vi "Format TBM.vi"(4 "WorkTable":refnum<class "WorkTable Class.lvclass">, 6 "Bond Pad Groups":T1[](array[typedef]), 7 "Inner/Outer":string, 8 "error in":errorcluster, 9 "Slot":i32, 10 "Chuck":i32, 11 "Console Log in":refnum<class "Console Log.lvclass">) -> (0 "error out":errorcluster, 2 "Formatted TBM":string[](array[string]), 3 "Console Log out":refnum<class "Console Log.lvclass">)   [LabVIEW 2011, in "Console Log.lvclass"]
uses:
  Console Log.lvclass
  Shared Components/Utils/Type Definitions/3d Line.ctl
  Shared Components/Vec3d Class/Vec3d Class.lvclass
  Shared Components/WorkTable Class/WorkTable Class.lvclass
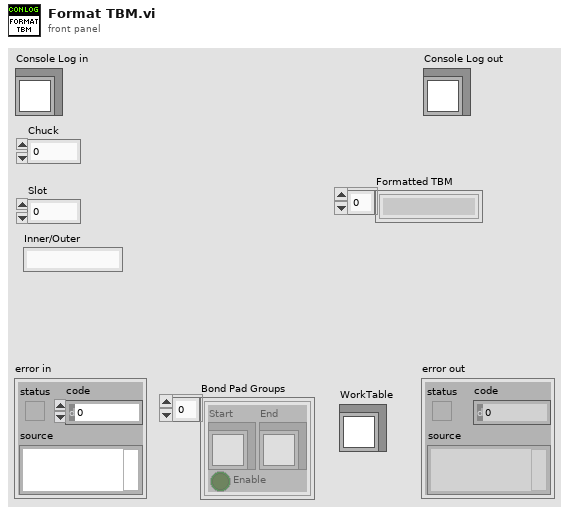
[diagram p1: front panel]
types:
  T1 = typedef "3d Line.ctl" = cluster{"Start":refnum<class "Vec3d Class.lvclass">, "End":refnum<class "Vec3d Class.lvclass">, "Enable":bool}
  T2 = typedef "Worktable_Module Slot.ctl" = cluster{"Slot State":enum16{"Empty", "Unglued", "Stamped", "PartOnTop", "Weighted", "Unpotted", "Potted"}, "BBM Type":enum16{"None", "BBM", "GlassSlide"}, "HDI Type":enum16{"None", "HDI", "Polyimide"}, "Vacuum Channel":u8, "Location/Orientation BBM":T3, "Location/Orientation HDI":T3, "S/N":string}
  T3 = typedef "Position_Orientation.ctl" = cluster{"Center":refnum<class "Vec3d Class.lvclass">, "Orientation":refnum<class "Orient3d Class.lvclass">}
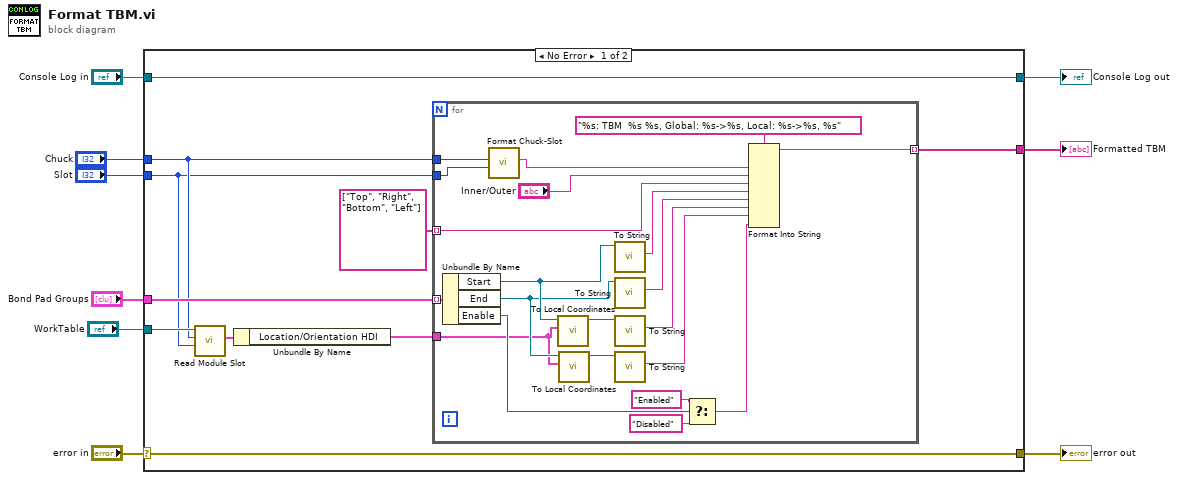
[diagram p0: block diagram]
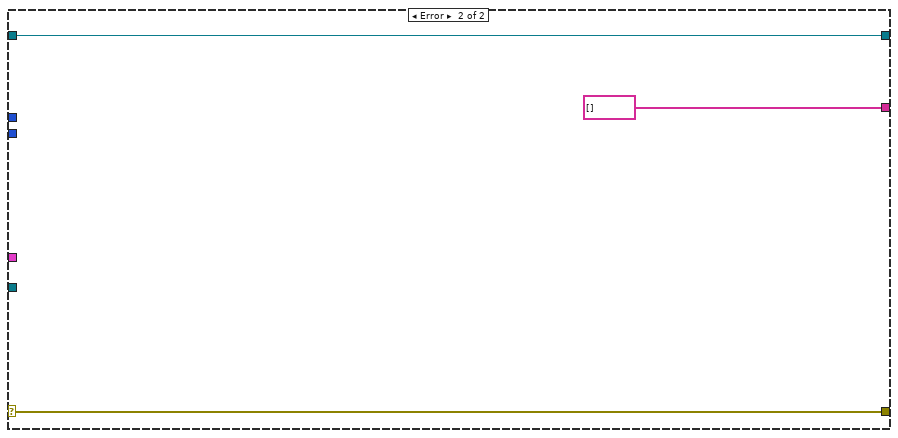
[diagram p2: hidden frame]
diagram:
  n1 = case shown="No Error" "error in" {
    selector: "error in" -> [w18 w43]
    tunnel: [w18 w43] -> w8
    tunnel: [w19 w42] -> w6
    tunnel: "Console Log in" -> [w19 w42]
    tunnel: "Bond Pad Groups" -> [w17 _]
    tunnel: [w16 string[] []] -> w4
    tunnel: "Chuck" -> [w13 _]
    tunnel: "Slot" -> [w12 _]
    tunnel: "WorkTable" -> [w14 _]
    frame No Error {
      n2 = call-dynamic "Read Module Slot.vi"("slot"=w12, "chuck"=w13, "WorkTable in"=w14) -> ("Module Slot"=w11:T2)  [unwired: 6 in, 2 out]
      n3 = Unbundle By Name(w11) -> ("Location/Orientation HDI"=w10:T3)
      n4 = for {
        tunnel: w17 -> [w40] mode=indexing
        tunnel: [w33] -> w16 mode=indexing
        tunnel: string[] ["Top", "Right", "Bottom", "Left"] -> [w31] mode=indexing
        tunnel: w13 -> [w22]
        tunnel: w12 -> [w21]
        tunnel: w10 -> [w23]
        n5 = Unbundle By Name(w40) -> ("Start"=w25:refnum<class "Vec3d Class.lvclass">, "End"=w24:refnum<class "Vec3d Class.lvclass">, "Enable"=w39:bool)
        n6 = call "Format Chuck-Slot.vi"("Slot"=w21, "Chuck"=w22) -> ("Formatted Chuck/Slot"=w20:string)  [unwired: 7 in, 2 out]
        n7 = call "To Local Coordinates.vi"("Center/Orientation"=w23, "Global Coordinates"=w25) -> ("Local Coordinates"=w30:refnum<class "Vec3d Class.lvclass">)  [unwired: 8 in, 1 out]
        n8 = call "To Local Coordinates.vi"("Center/Orientation"=w23, "Global Coordinates"=w24) -> ("Local Coordinates"=w29:refnum<class "Vec3d Class.lvclass">)  [unwired: 8 in, 1 out]
        n9 = call "To String.vi"("Vec3d in"=w25) -> ("Vec3d String"=w35:string)  [unwired: 8 in, 2 out]
        n10 = call "To String.vi"("Vec3d in"=w24) -> ("Vec3d String"=w34:string)  [unwired: 8 in, 2 out]
        n11 = call "To String.vi"("Vec3d in"=w30) -> ("Vec3d String"=w27:string)  [unwired: 8 in, 2 out]
        n12 = call "To String.vi"("Vec3d in"=w29) -> ("Vec3d String"=w26:string)  [unwired: 8 in, 2 out]
        n13 = Select(t="Enabled", s=w39, f="Disabled") -> (s? t:f=w28:string)
        n14 = Format Into String(format string="%s: TBM  %s %s, Global: %s->%s, Local: %s->%s, %s", w20, "Inner/Outer", w31, w35, w34, w27, w26, w28) -> (resulting string=w33:string)  [unwired: 2 in, 1 out]
      }
    }
    frame Error {
    }
  }
  "error out" <- w8
  "Console Log out" <- w6
  "Formatted TBM" <- w4
